vi "next state.vi"(7 "command":T2, 11 "actual state":T1) -> (3 "next state":T1)   [LabVIEW 2014]
doc: "This VI determines the next state.\n\n---------------------\npawlik@agh.edu.pl\n01.04.2019"
uses:
  command.ctl
  states.ctl
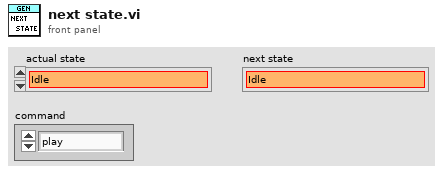
[diagram p1: front panel]
types:
  T1 = typedef "states.ctl" = enum16{"Idle", "Init", "Generate", "Stop", "Exit"}
  T2 = typedef "command.ctl" = enum16{"play", "stop", "exit"}
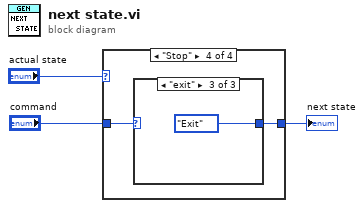
[diagram p0: block diagram]
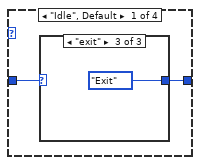
[diagram p2: hidden frame]
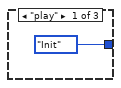
[diagram p3: hidden frame]
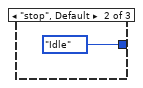
[diagram p4: hidden frame]
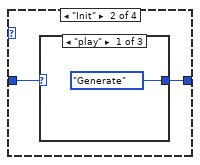
[diagram p5: hidden frame]
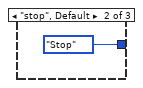
[diagram p6: hidden frame]
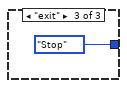
[diagram p7: hidden frame]
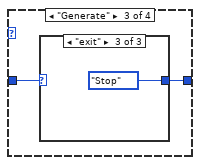
[diagram p8: hidden frame]
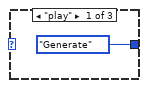
[diagram p9: hidden frame]
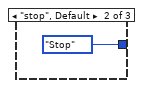
[diagram p10: hidden frame]
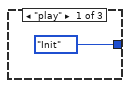
[diagram p11: hidden frame]
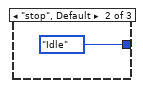
[diagram p12: hidden frame]
diagram:
  n1 = case shown="\"Stop\"" "actual state" {
    tunnel: "command" -> [w5 w10 w15 w20]
    tunnel: [w4 w9 w14 w19] -> w3
    frame "Idle", Default {
      n2 = case shown="\"exit\"" w5 {
        tunnel: [states."Init" ("Enum") states."Idle" ("Enum") states."Exit" ("Enum")] -> w4
        frame "play" {
        }
        frame "stop", Default {
        }
        frame "exit" {
        }
      }
    }
    frame "Init" {
      n3 = case shown="\"play\"" w10 {
        tunnel: [states."Generate" ("Enum") states."Stop" ("Enum") states."Stop" ("Enum")] -> w9
        frame "play" {
        }
        frame "stop", Default {
        }
        frame "exit" {
        }
      }
    }
    frame "Generate" {
      n4 = case shown="\"exit\"" w15 {
        tunnel: [states."Generate" ("Enum") states."Stop" ("Enum") states."Stop" ("Enum")] -> w14
        frame "play" {
        }
        frame "stop", Default {
        }
        frame "exit" {
        }
      }
    }
    frame "Stop" {
      n5 = case shown="\"exit\"" w20 {
        tunnel: [states."Init" ("Enum") states."Idle" ("Enum") states."Exit" ("Enum")] -> w19
        frame "play" {
        }
        frame "stop", Default {
        }
        frame "exit" {
        }
      }
    }
  }
  "next state" <- w3
